vi "SwissSPAD 1 Load FLI Dataset.vi"(5 "Image Type":string="Image", 8 "error in (no error)":errorcluster, 9 "Control References":T1, 10 "Folder Path":path, 11 "AlliGator IV DVR in":refnum<data-value>) -> (0 "error out":errorcluster, 2 "Folder Path (dup)":path, 3 "AlliGator IV DVR out":refnum<data-value>, 4 "Result String":string)   [LabVIEW 2021, in "SwissSPAD.lvlib"]
doc: "- - -\nAuthor: X. Michalet, Department of Chemistry & Biochemistry, UCLA\n(C) 2023, The Regents of the University of California"
uses:
  SwissSPAD.lvlib
  AlliGator/Files/AlliGator Files.lvlib
  <vilib>/vision/Image Controls.llb/IMAQ Image.ctl
  Phasor/Phasor Reference Series.ctl
  Phasor/Phasor.lvlib
  Phasor/Calibration Phasor (m, phi).ctl
  Phasor/Phasor (g, s).ctl
  Image/Named ROI Description.ctl
  Image/Image.lvlib
  AlliGator/Decay Analysis/Decay Preprocessing/AlliGator Baseline Subtraction Method.ctl
  AlliGator/Decay Analysis/Decay Preprocessing/AlliGator Decay Preprocessing.lvlib
  AlliGator/Decay Analysis/Decay Preprocessing/AlliGator Decay Background Subtraction Info.ctl
  AlliGator/Decay Analysis/Decay Preprocessing/AlliGator Decay Extrapolation Parameters.ctl
  AlliGator/Phasor Graph/AlliGator Decay Metadata v3.ctl
  AlliGator/Phasor Graph/AlliGator Phasor Graph.lvlib
  AlliGator/Phasor Graph/AlliGator Raw Phasor Plot Data v5.ctl
  AlliGator/Files/AlliGator Data Series Type.ctl
  AlliGator/Internal Variables/AlliGator Internal Variables v2.ctl
  AlliGator/Internal Variables/AlliGator Internal Variables.lvlib
  AlliGator/GUI/AlliGator Dataset Ctrl Refnums.ctl
  AlliGator/GUI/AlliGator GUI.lvlib
  AlliGator/Files/AlliGator FLI Dataset Type.ctl
  Phasor/Phasor Harmonic Data.ctl
  AlliGator/Phasor Plot/AlliGator Phasor Multi-Harmonic Data.ctl
  AlliGator/Phasor Plot/AlliGator Phasor Plot.lvlib
  AlliGator/Source Image/AlliGator Displayed Image.ctl
  AlliGator/Source Image/AlliGator Source Image.lvlib
  Fits/IRF(X)PSED/Decay Fit Parameters & Derived Quantities List v2.ctl
  Fits/Fits.lvlib
  Fits/IRF(X)PSED/Decay Fit Parameters In List.ctl
  AlliGator/Decay Analysis/Decay Fit/AlliGator Decay Fit Parameter Constraints 2.ctl
  AlliGator/Decay Analysis/Decay Fit/AlliGator Decay Fit.lvlib
  Fits/Decay Convolution/Decay Model.ctl
  Fits/Residual Type.ctl
  Fits/Fit Calculation Method.ctl
  Fits/Non-linear Fitting Algorithm.ctl
  AlliGator/Decay Fit Parameter Map/AlliGator Decay Fit Options & Parameters v3.ctl
  AlliGator/Decay Fit Parameter Map/AlliGator Decay Fit Parameter Map.lvlib
  Fits/IRF(X)PSED/Fit Weights Type.ctl
  AlliGator/Internal Variables/AlliGator Gate Image Set.ctl
  AlliGator/Settings/AlliGator Gate Arithmetic.ctl
  AlliGator/Settings/AlliGator Settings.lvlib
  AlliGator/Dual-Channel Datasets/AlliGator Dataset Channel.ctl
  AlliGator/Dual-Channel Datasets/AlliGator Dual-Channel Datasets.lvlib
  AlliGator/Decay Analysis/Decay Preprocessing/AlliGator Decay Preprocessing Parameters.ctl
  Graphs/XY Graph/XY Graph Plot Shift Method.ctl
  Graphs/XY Graph/XY Graph Add-Ons.lvlib
  Graphs/XY Graph/XY Graph Plot Shift Parameters.ctl
  Phasor/Phasor Standard Deviation Options.ctl
  Phasor/Phasor Calibration Map v2.ctl
  Fits/Non-linear Fitting Method v2.ctl
  Fits/IRF(X)PSED/MLE Baseline Offset Type.ctl
  AlliGator/Decay Fit Parameter Map/AlliGator Parameter Maps Data.ctl
  Fits/IRF(X)PSED/Decay Fit Options v3.ctl
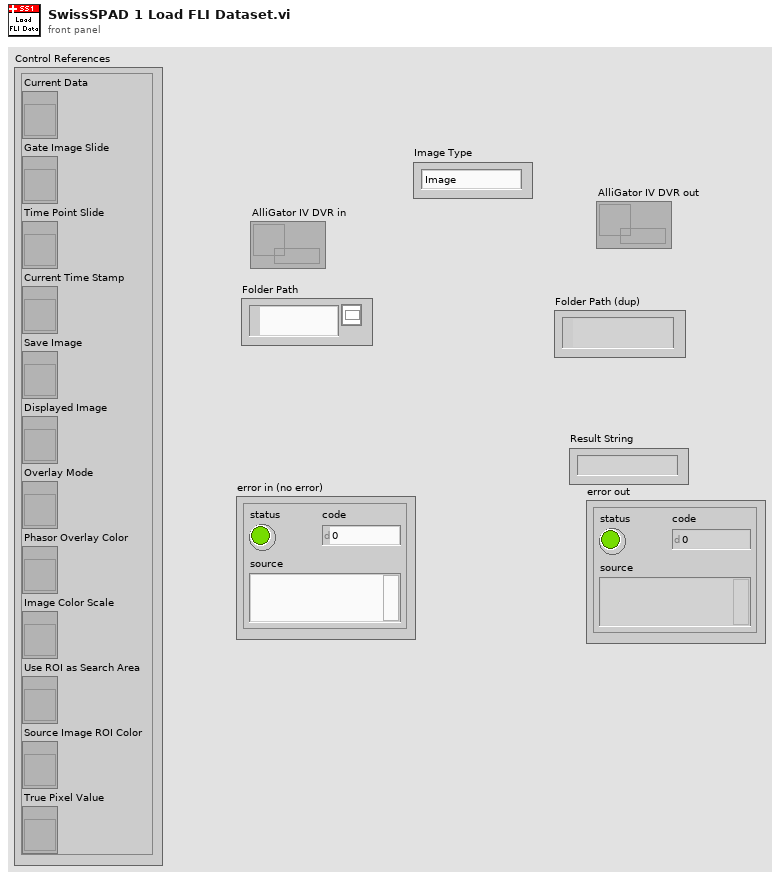
[diagram p1: front panel]
types:
  T1 = typedef "AlliGator GUI.lvlib/AlliGator Dataset Ctrl Refnums.ctl" = cluster{"Current Data":refnum<vi>, "Gate Image Slide":refnum<vi>, "Time Point Slide":refnum<vi>, "Current Time Stamp":refnum<vi>, "Save Image":refnum<vi>, "Displayed Image":refnum<vi>, "Overlay Mode":refnum<vi>, "Phasor Overlay Color":refnum<vi>, "Image Color Scale":refnum<vi>, "Use ROI as Search Area":refnum<vi>, "Source Image ROI Color":refnum<vi>, "True Pixel Value":refnum<vi>}
  T2 = typedef "AlliGator HDF5.lvlib/AlliGator FLI Data File Information.ctl" = cluster{"Load Single Gate Image VI Refnum":refnum<vi>, "File Info":variant, "FLI Parameters":T3, "FLI Dataset Type":T4}
  T3 = typedef "Phasor.lvlib/Phasor Fluorescence Lifetime Parameters v3.ctl" = cluster{"# Pixel X":i32, "# Pixel Y":i32, "# Gates":i32, "# Datasets":i32, "Gate Image Exposure":dbl[unit], "Macrotime Gate Separation":dbl[unit], "Nanotime Gate Separation":dbl[unit], "Gate Width":dbl[unit], "Laser Period":dbl[unit], "SYNC Period":dbl[unit], "Gate Image Integration":dbl[unit]}
  T4 = typedef "AlliGator Files.lvlib/AlliGator FLI Dataset Type.ctl" = enum16{"HDF5 FLI Dataset", "Gate Image Folder", ".sdt FLI Dataset (Becker & Hickl)", ".ptu FLI Dataset (PicoQuant)", "SS1 FLI Dataset", "SS2 FLI Dataset", "I/m/phi Dataset", ".bin FLI Dataset (PicoQuant Binned)", ".bin FLI Dataset (Piccolo Binned)", ".mat FLI Dataset"}
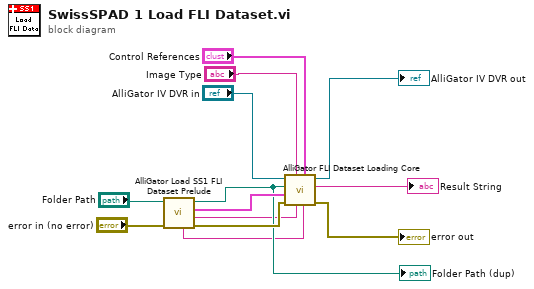
[diagram p0: block diagram]
diagram:
  n1 = call "AlliGator Load SS1 FLI Dataset Prelude.vi"("error in (no error)"="error in (no error)", "Path in"="Folder Path") -> ("error out"=w5:errorcluster, "Metadata"=w2:string, "FLI Data File Information"=w4:T2, "Path out"=w3:path, "Data Description"=w1:string)  [unwired: 5 in]
  "Folder Path (dup)" <- w3
  n2 = call "AlliGator FLI Dataset Loading Core.vi"("Data Description"=w1, "Control References"="Control References", "Metadata"=w2, "Image Type"="Image Type", "error in (no error)"=w5, "FLI Data File Information"=w4, "selected path"=w3, "Data Value Reference in"="AlliGator IV DVR in") -> ("error out"=→"error out":errorcluster, "Message"=→"Result String":string, "Data Value Reference out"=→"AlliGator IV DVR out":refnum<data-value>)  [unwired: 1 in]
